vi "Set State Display.vi"(4 "State":T1=enum."Initialising", 5 "error in (no error)":errorcluster) -> (0 "error out":errorcluster)   [LabVIEW 2023]
doc: "*-----------------------------------------------------\n* Author: SWatts\n*\n* VI Description: Sets the display dependent on State\n* \n*\n* Error handling: All errors passed out\n*\n* Pre-condition: \n*\n* Post-condition: None\n*\n* Revision History:\n*\n* Rev Date Author Description \n* 01 30/04/2014 SWatts First issue\n*\n*-----------------------------------------------------"
uses:
  Controls/DisplayQCommand.ctl
  Controls/DisplayMessage.ctl
  Controls/Tab.ctl
  Controls/SetupModeState.ctl
panel:
  # "Input"
  # "Output"
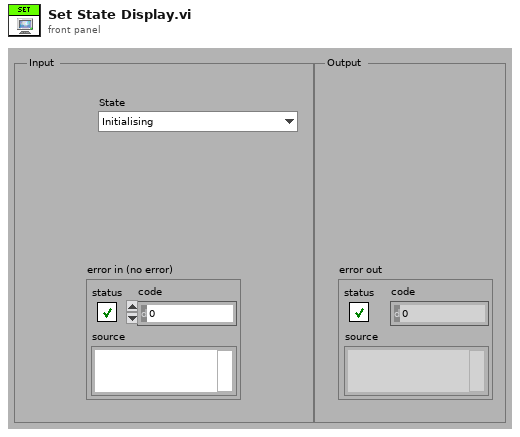
[diagram p1: front panel]
types:
  T1 = typedef "SetupModeState.ctl" = enum16{"No State - Error", "Initialising", "Idling", "Running", "Sorting Menu", "Resetting Menu", "Loading UI", "Erroring", "Exiting"}
  T2 = typedef "Tab.ctl" = enum32{"Welcome Screen", "Eng Set Up", "Oppo Run Screen", "Eng Run Screen", "Test Report Screen", "Error"}
  T3 = typedef "DisplayMessage.ctl" = enum16{"No Message - Ignore", "Display Message", "Set Tab", "Set Status", "Add Error Message", "Clear Error History", "Generate Error", "Set Idling Display", "Set Running Display", "Set Subpanel Output", "Stop"}
  T4 = typedef "DisplayQCommand.ctl" = enum16{"No Command - Error", "Initialise", "Get Q Reference", "Add Item to Bottom", "Add Item to Top", "Flush Q", "Dequeue", "Peek Next Element", "Close"}
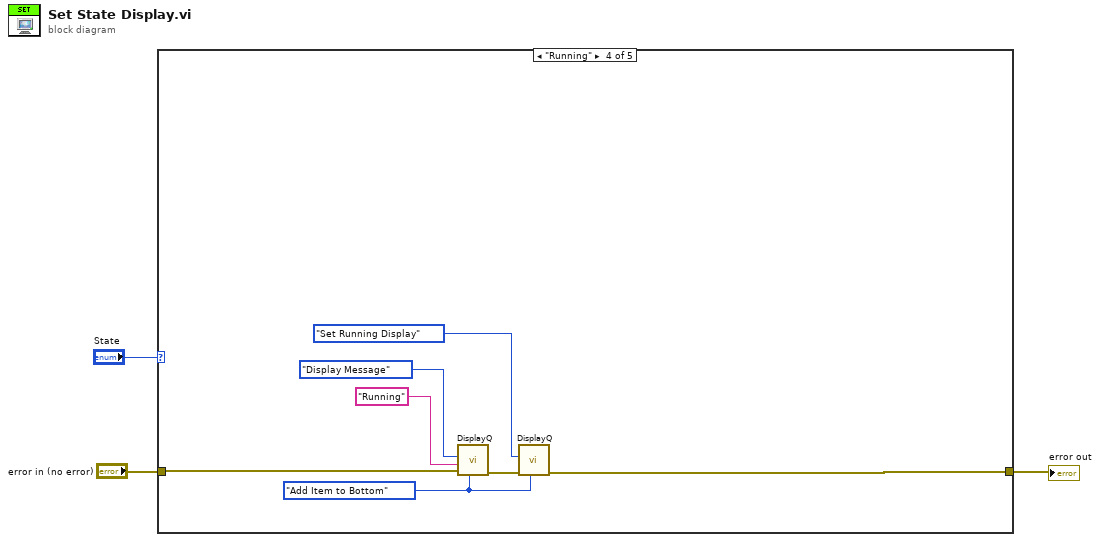
[diagram p0: block diagram]
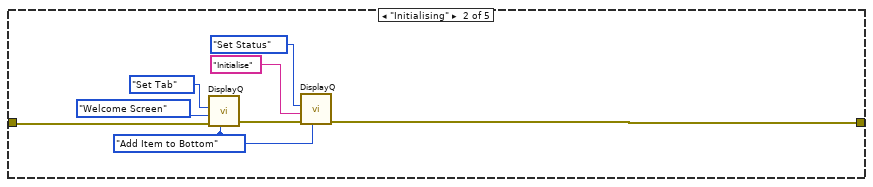
[diagram p3: hidden frame]
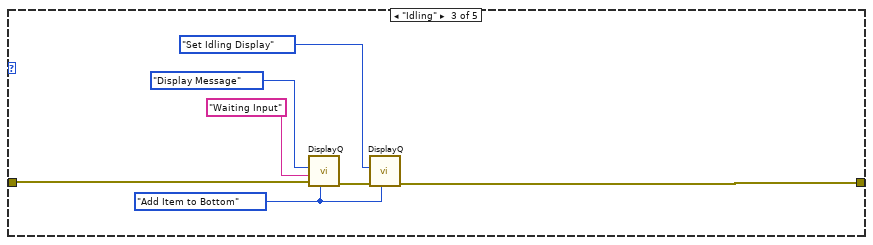
[diagram p4: hidden frame]
diagram:
  n1 = case shown="\"Running\"" "State" {
    tunnel: "error in (no error)" -> [w4 w12 w17 w24 w27]
    tunnel: [w4 w6 w14 w21 w27] -> w1
    frame "No State - Error", Default {
    }
    frame "Initialising" {
      w7 = DisplayQCommand."Add Item to Bottom" ("command")
      n2 = call "DisplayQ.vi"("command"=w7, "error in (no error)"=w12, "DataIn"=Tab."Welcome Screen" ("Tab Control"), "DisplayMessage"=DisplayMessage."Set Tab") -> ("error out"=w8:errorcluster)  [unwired: 1 in, 3 out]
      n3 = call "DisplayQ.vi"("command"=w7, "error in (no error)"=w8, "DataIn"="Initialise", "DisplayMessage"=DisplayMessage."Set Status") -> ("error out"=w6:errorcluster)  [unwired: 1 in, 3 out]
    }
    frame "Idling" {
      w15 = DisplayQCommand."Add Item to Bottom" ("command")
      n4 = call "DisplayQ.vi"("command"=w15, "error in (no error)"=w17, "DataIn"="Waiting Input", "DisplayMessage"=DisplayMessage."Display Message") -> ("error out"=w16:errorcluster)  [unwired: 1 in, 3 out]
      n5 = call "DisplayQ.vi"("command"=w15, "error in (no error)"=w16, "DisplayMessage"=DisplayMessage."Set Idling Display") -> ("error out"=w14:errorcluster)  [unwired: 2 in, 3 out]
    }
    frame "Running" {
      w22 = DisplayQCommand."Add Item to Bottom" ("command")
      n6 = call "DisplayQ.vi"("command"=w22, "error in (no error)"=w24, "DataIn"="Running", "DisplayMessage"=DisplayMessage."Display Message") -> ("error out"=w23:errorcluster)  [unwired: 1 in, 3 out]
      n7 = call "DisplayQ.vi"("command"=w22, "error in (no error)"=w23, "DisplayMessage"=DisplayMessage."Set Running Display") -> ("error out"=w21:errorcluster)  [unwired: 2 in, 3 out]
    }
    frame "Erroring" {
    }
  }
  "error out" <- w1
